vi "Untitled 2.vi"(8 "error in (no error)":errorcluster, 11 "LineCCD in":refnum<class "LineCCD.lvclass">) -> (0 "error out":errorcluster, 3 "LineCCD out":refnum<class "LineCCD.lvclass">)   [LabVIEW 2012, in "LineCCD.lvclass"]
uses:
  LineCCD.lvclass
  LineCCD.lvclass/LineCCD.ctl
panel:
  out "x/y":dbl
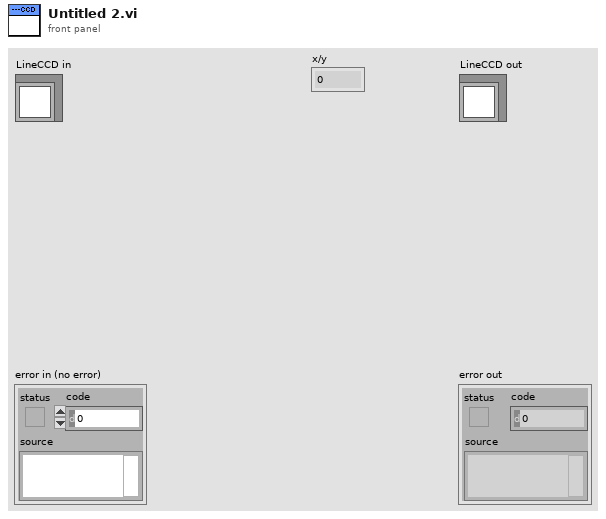
[diagram p1: front panel]
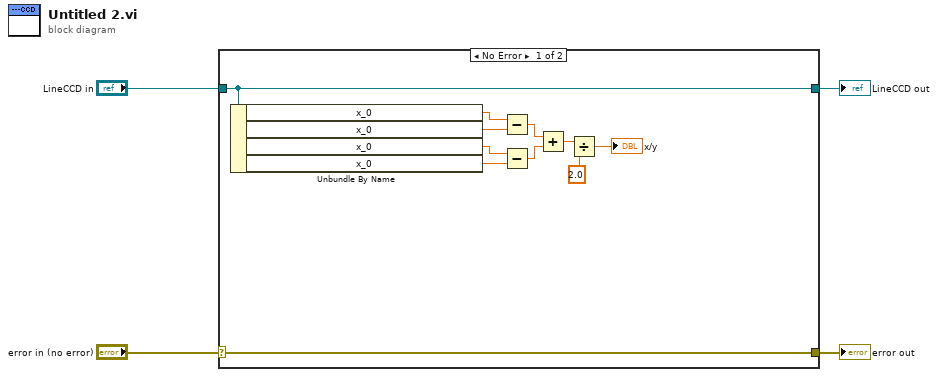
[diagram p0: block diagram]
diagram:
  n1 = case shown="No Error" "error in (no error)" {
    selector: "error in (no error)" -> [w15 w17]
    tunnel: [w15 w17] -> w3
    tunnel: [w14 w16] -> w1
    tunnel: "LineCCD in" -> [w14 w16]
    frame No Error {
      n2 = Unbundle By Name(w14) -> ("x_0"=w13:dbl, "x_0"=w12:dbl, "x_0"=w11:dbl, "x_0"=w10:dbl)
      n3 = Subtract(x=w13, y=w12) -> (x-y=w9:dbl)
      n4 = Subtract(x=w11, y=w10) -> (x-y=w8:dbl)
      n5 = Add(x=w9, y=w8) -> (x+y=w7:dbl)
      n6 = Divide(x=w7, y=2.0) -> (x/y=→"x/y":dbl)
    }
    frame Error {
    }
  }
  "error out" <- w3
  "LineCCD out" <- w1
